vi "S4GUI_001.vi"() -> ()   [LabVIEW 2018] (continued)
        n2695 = call-dynamic "Write Kinetic Series Length.vi"("error in (no error)"=w6553, "Kinetic Series Length"=w6544, "Interface in"=w6554) -> ("error out"=w6545:errorcluster, "Interface out"=w6546:refnum<class "Interface.lvclass">)  [unwired: 7 in]
        n2696 = call-dynamic "Write Interface.vi"("error in (no error)"=w6545, "Interface.lvclass"=w6546, "Channel in"=w6552) -> ("error out"=w6551:errorcluster, "Channel out"=w6550:refnum<class "Channel.lvclass">)  [unwired: 7 in]
        n2697 = call-dynamic "Write Channel.vi"("error in (no error)"=w6551, "Channel.lvclass"=w6550, "Acquisition in"=w6549) -> ("error out"=w6555:errorcluster, "Acquisition out"=w6557:refnum<class "Acquisition.lvclass">)  [unwired: 7 in]
        n2698 = call-dynamic "Write AcquisitionA.vi"("error in (no error)"=w6555, "Acquisition.lvclass"=w6557, "S4ACS_GUI in"=w6556) -> ("error out"=w6541:errorcluster, "S4ACS_GUI out"=w6540:refnum<class "S4GUI.lvclass">)  [unwired: 7 in]
      }
      event "Stop ch1": Value Change {
        n2699 = event-data() -> ()  [unwired: 1 in, 6 out]
        n2700 = disable-structure shown="Enabled" {
          disable-tunnel: w6563 -> [w6596 w6624]
          disable-tunnel: w6562 -> [w6594 w6617]
          disable-tunnel: [w6576 w6616] -> w6561
          disable-tunnel: [w6564 w6624] -> w6560
          frame Disabled {
            # "Para movimento \nda lamina retardadora"
            # "Restaura a última sequência de lâminas"
            n2701 = call-dynamic "Read AcquisitionA.vi"("error in (no error)"=w6594, "S4ACS_GUI in"=w6596) -> ("error out"=w6598:errorcluster, "Acquisition.lvclass"=w6597:refnum<class "Acquisition.lvclass">, "S4ACS_GUI out"=w6595:refnum<class "S4GUI.lvclass">)  [unwired: 7 in]
            n2702 = disable-structure shown="Enabled" {
              disable-tunnel: w6598 -> [w6603 w6614]
              disable-tunnel: w6597 -> [w6602 w6615]
              disable-tunnel: [w6600 w6615] -> w6592
              disable-tunnel: [w6599 w6614] -> w6591
              frame Disabled {
                # "Só precisa enviar comando STOP quando\no controle dos ciclos for feito pelo ACS."
                n2703 = call-dynamic "Read Channel.vi"("error in (no error)"=w6603, "Acquisition in"=w6602) -> ("error out"=w6605:errorcluster, "Channel.lvclass"=w6604:refnum<class "Channel.lvclass">, "Acquisition out"=w6611:refnum<class "Acquisition.lvclass">)  [unwired: 7 in]
                n2704 = call-dynamic "Read State Machine.vi"("error in (no error)"=w6605, "Device in"=w6604) -> ("error out"=w6607:errorcluster, "State Machine.lvclass"=w6606:refnum<class "State Machine.lvclass">, "Device out"=w6609:refnum<class "Channel.lvclass">)  [unwired: 7 in]
                n2705 = call "Next State.vi"("error in (no error)"=w6607, "New_State"=u32 70, "State Machine in"=w6606) -> ("error out"=w6610:errorcluster, "State Machine out"=w6608:refnum<class "State Machine.lvclass">)  [unwired: 7 in]
                n2706 = call-dynamic "Write State Machine.vi"("error in (no error)"=w6610, "State Machine.lvclass"=w6608, "Device in"=w6609) -> ("error out"=w6612:errorcluster, "Device out"=w6613:refnum<class "Channel.lvclass">)  [unwired: 7 in]
                n2707 = call-dynamic "Write Channel.vi"("error in (no error)"=w6612, "Channel.lvclass"=w6613, "Acquisition in"=w6611) -> ("error out"=w6599:errorcluster, "Acquisition out"=w6600:refnum<class "Acquisition.lvclass">)  [unwired: 7 in]
              }
              frame Enabled {
                # "Não precisa enviar comando STOP para o ACS\nenquanto o controle dos ciclos for feito pela GUI."
              }
            }
            n2708 = call-dynamic "Write Acq_state.vi"("error in (no error)"=w6591, "Acq_state"=u32 0, "Acquisition in"=w6592) -> ("error out"=w6590:errorcluster, "Acquisition out"=w6589:refnum<class "Acquisition.lvclass">)  [unwired: 7 in]
            n2709 = call-dynamic "Write AcquisitionA.vi"("error in (no error)"=w6590, "Acquisition.lvclass"=w6589, "S4ACS_GUI in"=w6595) -> ("error out"=w6577:errorcluster, "S4ACS_GUI out"=w6575:refnum<class "S4GUI.lvclass">)  [unwired: 7 in]
            n2710 = call "Read Instrument.lvclass.vi"("error in (no error)"=w6577, "S4ACS_GUI in"=w6575) -> ("error out"=w6584:errorcluster, "Instrument.lvclass"=w6587:refnum<class "Instrument.lvclass">, "S4ACS_GUI out"=w6588:refnum<class "S4GUI.lvclass">)  [unwired: 7 in]
            n2711 = call "Read WPROT.vi"("error in (no error)"=w6584, "Instrument in"=w6587) -> ("error out"=w6583:errorcluster, "Opt_Selector.lvclass"=w6585:refnum<class "Opt_Selector.lvclass">, "Instrument out"=w6586:refnum<class "Instrument.lvclass">)  [unwired: 7 in]
            n2712 = call-dynamic "Read sequencia_ant.vi"("error in (no error)"=w6583, "Opt_Selector in"=w6585) -> ("error out"=w6579:errorcluster, "sequencia_ant"=w6578:u16, "Opt_Selector out"=w6580:refnum<class "Opt_Selector.lvclass">)  [unwired: 7 in]
            n2713 = call-dynamic "Write sequencia.vi"("error in (no error)"=w6579, "sequencia"=w6578, "Opt_Selector in"=w6580) -> ("error out"=w6566:errorcluster, "Opt_Selector out"=w6569:refnum<class "Opt_Selector.lvclass">)  [unwired: 7 in]
            n2714 = call-dynamic "Read State Machine.vi"("error in (no error)"=w6566, "Device in"=w6569) -> ("error out"=w6571:errorcluster, "State Machine.lvclass"=w6574:refnum<class "State Machine.lvclass">, "Device out"=w6568:refnum<class "Opt_Selector.lvclass">)  [unwired: 7 in]
            n2715 = call "Next State.vi"("error in (no error)"=w6571, "New_State"=10, "State Machine in"=w6574) -> ("error out"=w6570:errorcluster, "State Machine out"=w6573:refnum<class "State Machine.lvclass">)  [unwired: 7 in]
            n2716 = call-dynamic "Write State Machine.vi"("error in (no error)"=w6570, "State Machine.lvclass"=w6573, "Device in"=w6568) -> ("error out"=w6565:errorcluster, "Device out"=w6567:refnum<class "Opt_Selector.lvclass">)  [unwired: 7 in]
            n2717 = call "Write WPROT.vi"("error in (no error)"=w6565, "Opt_Selector.lvclass"=w6567, "Instrument in"=w6586) -> ("error out"=w6582:errorcluster, "Instrument out"=w6581:refnum<class "Instrument.lvclass">)  [unwired: 7 in]
            n2718 = call "Write Instrument.lvclass.vi"("error in (no error)"=w6582, "Instrument.lvclass"=w6581, "S4ACS_GUI in"=w6588) -> ("error out"=w6576:errorcluster, "S4ACS_GUI out"=w6564:refnum<class "S4GUI.lvclass">)  [unwired: 7 in]
          }
          frame Enabled {
            w6619 = FALSE ("Wait Until Done")
            n2719 = call <vilib>:"Application Directory.vi"() -> ("Application Directory"=w6622:path)
            n2720 = Build Path(base path=w6622, name or relative path="MsgStop1.vi") -> (appended path=w6623:path)
            n2721 = Open VI Reference(vi path=w6623, error in (no error)=w6617) -> (vi reference=w6621:refnum<vi>, error out=w6620:errorcluster)  [unwired: 4 in]
            n2722 = invoke class="VI" method="Run VI"(reference=w6621, error in=w6620, "Wait until done"=w6619, "Auto Dispose Ref"=w6619) -> (error out=w6616:errorcluster)  [unwired: 1 in, 4 out]
          }
        }
      }
      event "Stop ch2": Value Change {
        n2723 = event-data() -> ()  [unwired: 1 in, 6 out]
        n2724 = disable-structure shown="Enabled" {
          disable-tunnel: w6628 -> [w6661 w6681]
          disable-tunnel: w6627 -> [w6659 w6683]
          disable-tunnel: [w6641 w6682] -> w6626
          disable-tunnel: [w6629 w6681] -> w6625
          frame Disabled {
            # "Para movimento \nda lamina retardadora"
            # "Restaura a última sequência de lâminas"
            n2725 = call "Read AcquisitionB.vi"("error in (no error)"=w6659, "S4ACS_GUI in"=w6661) -> ("error out"=w6663:errorcluster, "Acquisition.lvclass"=w6662:refnum<class "Acquisition.lvclass">, "S4ACS_GUI out"=w6660:refnum<class "S4GUI.lvclass">)  [unwired: 7 in]
            n2726 = disable-structure shown="Enabled" {
              disable-tunnel: w6663 -> [w6668 w6679]
              disable-tunnel: w6662 -> [w6667 w6680]
              disable-tunnel: [w6665 w6680] -> w6657
              disable-tunnel: [w6664 w6679] -> w6656
              frame Disabled {
                # "Só precisa enviar comando STOP quando\no controle dos ciclos for feito pelo ACS."
                n2727 = call-dynamic "Read Channel.vi"("error in (no error)"=w6668, "Acquisition in"=w6667) -> ("error out"=w6670:errorcluster, "Channel.lvclass"=w6669:refnum<class "Channel.lvclass">, "Acquisition out"=w6676:refnum<class "Acquisition.lvclass">)  [unwired: 7 in]
                n2728 = call-dynamic "Read State Machine.vi"("error in (no error)"=w6670, "Device in"=w6669) -> ("error out"=w6672:errorcluster, "State Machine.lvclass"=w6671:refnum<class "State Machine.lvclass">, "Device out"=w6674:refnum<class "Channel.lvclass">)  [unwired: 7 in]
                n2729 = call "Next State.vi"("error in (no error)"=w6672, "New_State"=u32 70, "State Machine in"=w6671) -> ("error out"=w6675:errorcluster, "State Machine out"=w6673:refnum<class "State Machine.lvclass">)  [unwired: 7 in]
                n2730 = call-dynamic "Write State Machine.vi"("error in (no error)"=w6675, "State Machine.lvclass"=w6673, "Device in"=w6674) -> ("error out"=w6677:errorcluster, "Device out"=w6678:refnum<class "Channel.lvclass">)  [unwired: 7 in]
                n2731 = call-dynamic "Write Channel.vi"("error in (no error)"=w6677, "Channel.lvclass"=w6678, "Acquisition in"=w6676) -> ("error out"=w6664:errorcluster, "Acquisition out"=w6665:refnum<class "Acquisition.lvclass">)  [unwired: 7 in]
              }
              frame Enabled {
                # "Não precisa enviar comando STOP para o ACS\nenquanto o controle dos ciclos for feito pela GUI."
              }
            }
            n2732 = call-dynamic "Write Acq_state.vi"("error in (no error)"=w6656, "Acq_state"=u32 0, "Acquisition in"=w6657) -> ("error out"=w6655:errorcluster, "Acquisition out"=w6654:refnum<class "Acquisition.lvclass">)  [unwired: 7 in]
            n2733 = call "Write AcquisitionB.vi"("error in (no error)"=w6655, "Acquisition.lvclass"=w6654, "S4ACS_GUI in"=w6660) -> ("error out"=w6642:errorcluster, "S4ACS_GUI out"=w6640:refnum<class "S4GUI.lvclass">)  [unwired: 7 in]
            n2734 = call "Read Instrument.lvclass.vi"("error in (no error)"=w6642, "S4ACS_GUI in"=w6640) -> ("error out"=w6649:errorcluster, "Instrument.lvclass"=w6652:refnum<class "Instrument.lvclass">, "S4ACS_GUI out"=w6653:refnum<class "S4GUI.lvclass">)  [unwired: 7 in]
            n2735 = call "Read WPROT.vi"("error in (no error)"=w6649, "Instrument in"=w6652) -> ("error out"=w6648:errorcluster, "Opt_Selector.lvclass"=w6650:refnum<class "Opt_Selector.lvclass">, "Instrument out"=w6651:refnum<class "Instrument.lvclass">)  [unwired: 7 in]
            n2736 = call-dynamic "Read sequencia_ant.vi"("error in (no error)"=w6648, "Opt_Selector in"=w6650) -> ("error out"=w6644:errorcluster, "sequencia_ant"=w6643:u16, "Opt_Selector out"=w6645:refnum<class "Opt_Selector.lvclass">)  [unwired: 7 in]
            n2737 = call-dynamic "Write sequencia.vi"("error in (no error)"=w6644, "sequencia"=w6643, "Opt_Selector in"=w6645) -> ("error out"=w6631:errorcluster, "Opt_Selector out"=w6634:refnum<class "Opt_Selector.lvclass">)  [unwired: 7 in]
            n2738 = call-dynamic "Read State Machine.vi"("error in (no error)"=w6631, "Device in"=w6634) -> ("error out"=w6636:errorcluster, "State Machine.lvclass"=w6639:refnum<class "State Machine.lvclass">, "Device out"=w6633:refnum<class "Opt_Selector.lvclass">)  [unwired: 7 in]
            n2739 = call "Next State.vi"("error in (no error)"=w6636, "New_State"=10, "State Machine in"=w6639) -> ("error out"=w6635:errorcluster, "State Machine out"=w6638:refnum<class "State Machine.lvclass">)  [unwired: 7 in]
            n2740 = call-dynamic "Write State Machine.vi"("error in (no error)"=w6635, "State Machine.lvclass"=w6638, "Device in"=w6633) -> ("error out"=w6630:errorcluster, "Device out"=w6632:refnum<class "Opt_Selector.lvclass">)  [unwired: 7 in]
            n2741 = call "Write WPROT.vi"("error in (no error)"=w6630, "Opt_Selector.lvclass"=w6632, "Instrument in"=w6651) -> ("error out"=w6647:errorcluster, "Instrument out"=w6646:refnum<class "Instrument.lvclass">)  [unwired: 7 in]
            n2742 = call "Write Instrument.lvclass.vi"("error in (no error)"=w6647, "Instrument.lvclass"=w6646, "S4ACS_GUI in"=w6653) -> ("error out"=w6641:errorcluster, "S4ACS_GUI out"=w6629:refnum<class "S4GUI.lvclass">)  [unwired: 7 in]
          }
          frame Enabled {
            w6685 = FALSE ("Wait Until Done")
            n2743 = call <vilib>:"Application Directory.vi"() -> ("Application Directory"=w6688:path)
            n2744 = Build Path(base path=w6688, name or relative path="MsgStop2.vi") -> (appended path=w6689:path)
            n2745 = Open VI Reference(vi path=w6689, error in (no error)=w6683) -> (vi reference=w6687:refnum<vi>, error out=w6686:errorcluster)  [unwired: 4 in]
            n2746 = invoke class="VI" method="Run VI"(reference=w6687, error in=w6686, "Wait until done"=w6685, "Auto Dispose Ref"=w6685) -> (error out=w6682:errorcluster)  [unwired: 1 in, 4 out]
          }
        }
      }
      event "Stop ch3": Value Change {
        n2747 = event-data() -> ()  [unwired: 1 in, 6 out]
        n2748 = disable-structure shown="Enabled" {
          disable-tunnel: w6693 -> [w6726 w6746]
          disable-tunnel: w6692 -> [w6724 w6748]
          disable-tunnel: [w6706 w6747] -> w6691
          disable-tunnel: [w6694 w6746] -> w6690
          frame Disabled {
            # "Para movimento \nda lamina retardadora"
            # "Restaura a última sequência de lâminas"
            n2749 = call-dynamic "Read AcquisitionC.vi"("error in (no error)"=w6724, "S4ACS_GUI in"=w6726) -> ("error out"=w6728:errorcluster, "Acquisition.lvclass"=w6727:refnum<class "Acquisition.lvclass">, "S4ACS_GUI out"=w6725:refnum<class "S4GUI.lvclass">)  [unwired: 7 in]
            n2750 = disable-structure shown="Enabled" {
              disable-tunnel: w6728 -> [w6733 w6744]
              disable-tunnel: w6727 -> [w6732 w6745]
              disable-tunnel: [w6730 w6745] -> w6722
              disable-tunnel: [w6729 w6744] -> w6721
              frame Disabled {
                # "Só precisa enviar comando STOP quando\no controle dos ciclos for feito pelo ACS."
                n2751 = call-dynamic "Read Channel.vi"("error in (no error)"=w6733, "Acquisition in"=w6732) -> ("error out"=w6735:errorcluster, "Channel.lvclass"=w6734:refnum<class "Channel.lvclass">, "Acquisition out"=w6741:refnum<class "Acquisition.lvclass">)  [unwired: 7 in]
                n2752 = call-dynamic "Read State Machine.vi"("error in (no error)"=w6735, "Device in"=w6734) -> ("error out"=w6737:errorcluster, "State Machine.lvclass"=w6736:refnum<class "State Machine.lvclass">, "Device out"=w6739:refnum<class "Channel.lvclass">)  [unwired: 7 in]
                n2753 = call "Next State.vi"("error in (no error)"=w6737, "New_State"=u32 70, "State Machine in"=w6736) -> ("error out"=w6740:errorcluster, "State Machine out"=w6738:refnum<class "State Machine.lvclass">)  [unwired: 7 in]
                n2754 = call-dynamic "Write State Machine.vi"("error in (no error)"=w6740, "State Machine.lvclass"=w6738, "Device in"=w6739) -> ("error out"=w6742:errorcluster, "Device out"=w6743:refnum<class "Channel.lvclass">)  [unwired: 7 in]
                n2755 = call-dynamic "Write Channel.vi"("error in (no error)"=w6742, "Channel.lvclass"=w6743, "Acquisition in"=w6741) -> ("error out"=w6729:errorcluster, "Acquisition out"=w6730:refnum<class "Acquisition.lvclass">)  [unwired: 7 in]
              }
              frame Enabled {
                # "Não precisa enviar comando STOP para o ACS\nenquanto o controle dos ciclos for feito pela GUI."
              }
            }
            n2756 = call-dynamic "Write Acq_state.vi"("error in (no error)"=w6721, "Acq_state"=u32 0, "Acquisition in"=w6722) -> ("error out"=w6720:errorcluster, "Acquisition out"=w6719:refnum<class "Acquisition.lvclass">)  [unwired: 7 in]
            n2757 = call-dynamic "Write AcquisitionC.vi"("error in (no error)"=w6720, "Acquisition.lvclass"=w6719, "S4ACS_GUI in"=w6725) -> ("error out"=w6707:errorcluster, "S4ACS_GUI out"=w6705:refnum<class "S4GUI.lvclass">)  [unwired: 7 in]
            n2758 = call "Read Instrument.lvclass.vi"("error in (no error)"=w6707, "S4ACS_GUI in"=w6705) -> ("error out"=w6714:errorcluster, "Instrument.lvclass"=w6717:refnum<class "Instrument.lvclass">, "S4ACS_GUI out"=w6718:refnum<class "S4GUI.lvclass">)  [unwired: 7 in]
            n2759 = call "Read WPROT.vi"("error in (no error)"=w6714, "Instrument in"=w6717) -> ("error out"=w6713:errorcluster, "Opt_Selector.lvclass"=w6715:refnum<class "Opt_Selector.lvclass">, "Instrument out"=w6716:refnum<class "Instrument.lvclass">)  [unwired: 7 in]
            n2760 = call-dynamic "Read sequencia_ant.vi"("error in (no error)"=w6713, "Opt_Selector in"=w6715) -> ("error out"=w6709:errorcluster, "sequencia_ant"=w6708:u16, "Opt_Selector out"=w6710:refnum<class "Opt_Selector.lvclass">)  [unwired: 7 in]
            n2761 = call-dynamic "Write sequencia.vi"("error in (no error)"=w6709, "sequencia"=w6708, "Opt_Selector in"=w6710) -> ("error out"=w6696:errorcluster, "Opt_Selector out"=w6699:refnum<class "Opt_Selector.lvclass">)  [unwired: 7 in]
            n2762 = call-dynamic "Read State Machine.vi"("error in (no error)"=w6696, "Device in"=w6699) -> ("error out"=w6701:errorcluster, "State Machine.lvclass"=w6704:refnum<class "State Machine.lvclass">, "Device out"=w6698:refnum<class "Opt_Selector.lvclass">)  [unwired: 7 in]
            n2763 = call "Next State.vi"("error in (no error)"=w6701, "New_State"=10, "State Machine in"=w6704) -> ("error out"=w6700:errorcluster, "State Machine out"=w6703:refnum<class "State Machine.lvclass">)  [unwired: 7 in]
            n2764 = call-dynamic "Write State Machine.vi"("error in (no error)"=w6700, "State Machine.lvclass"=w6703, "Device in"=w6698) -> ("error out"=w6695:errorcluster, "Device out"=w6697:refnum<class "Opt_Selector.lvclass">)  [unwired: 7 in]
            n2765 = call "Write WPROT.vi"("error in (no error)"=w6695, "Opt_Selector.lvclass"=w6697, "Instrument in"=w6716) -> ("error out"=w6712:errorcluster, "Instrument out"=w6711:refnum<class "Instrument.lvclass">)  [unwired: 7 in]
            n2766 = call "Write Instrument.lvclass.vi"("error in (no error)"=w6712, "Instrument.lvclass"=w6711, "S4ACS_GUI in"=w6718) -> ("error out"=w6706:errorcluster, "S4ACS_GUI out"=w6694:refnum<class "S4GUI.lvclass">)  [unwired: 7 in]
          }
          frame Enabled {
            w6750 = FALSE ("Wait Until Done")
            n2767 = call <vilib>:"Application Directory.vi"() -> ("Application Directory"=w6753:path)
            n2768 = Build Path(base path=w6753, name or relative path="MsgStop3.vi") -> (appended path=w6754:path)
            n2769 = Open VI Reference(vi path=w6754, error in (no error)=w6748) -> (vi reference=w6752:refnum<vi>, error out=w6751:errorcluster)  [unwired: 4 in]
            n2770 = invoke class="VI" method="Run VI"(reference=w6752, error in=w6751, "Wait until done"=w6750, "Auto Dispose Ref"=w6750) -> (error out=w6747:errorcluster)  [unwired: 1 in, 4 out]
          }
        }
      }
      event "Stop ch4": Value Change {
        n2771 = event-data() -> ()  [unwired: 1 in, 6 out]
        n2772 = disable-structure shown="Enabled" {
          disable-tunnel: w6758 -> [w6791 w6811]
          disable-tunnel: w6757 -> [w6789 w6813]
          disable-tunnel: [w6771 w6812] -> w6756
          disable-tunnel: [w6759 w6811] -> w6755
          frame Disabled {
            # "Para movimento \nda lamina retardadora"
            # "Restaura a última sequência de lâminas"
            n2773 = call-dynamic "Read AcquisitionD.vi"("error in (no error)"=w6789, "S4ACS_GUI in"=w6791) -> ("error out"=w6793:errorcluster, "Acquisition.lvclass"=w6792:refnum<class "Acquisition.lvclass">, "S4ACS_GUI out"=w6790:refnum<class "S4GUI.lvclass">)  [unwired: 7 in]
            n2774 = disable-structure shown="Enabled" {
              disable-tunnel: w6793 -> [w6798 w6809]
              disable-tunnel: w6792 -> [w6797 w6810]
              disable-tunnel: [w6795 w6810] -> w6787
              disable-tunnel: [w6794 w6809] -> w6786
              frame Disabled {
                # "Só precisa enviar comando STOP quando\no controle dos ciclos for feito pelo ACS."
                n2775 = call-dynamic "Read Channel.vi"("error in (no error)"=w6798, "Acquisition in"=w6797) -> ("error out"=w6800:errorcluster, "Channel.lvclass"=w6799:refnum<class "Channel.lvclass">, "Acquisition out"=w6806:refnum<class "Acquisition.lvclass">)  [unwired: 7 in]
                n2776 = call-dynamic "Read State Machine.vi"("error in (no error)"=w6800, "Device in"=w6799) -> ("error out"=w6802:errorcluster, "State Machine.lvclass"=w6801:refnum<class "State Machine.lvclass">, "Device out"=w6804:refnum<class "Channel.lvclass">)  [unwired: 7 in]
                n2777 = call "Next State.vi"("error in (no error)"=w6802, "New_State"=u32 70, "State Machine in"=w6801) -> ("error out"=w6805:errorcluster, "State Machine out"=w6803:refnum<class "State Machine.lvclass">)  [unwired: 7 in]
                n2778 = call-dynamic "Write State Machine.vi"("error in (no error)"=w6805, "State Machine.lvclass"=w6803, "Device in"=w6804) -> ("error out"=w6807:errorcluster, "Device out"=w6808:refnum<class "Channel.lvclass">)  [unwired: 7 in]
                n2779 = call-dynamic "Write Channel.vi"("error in (no error)"=w6807, "Channel.lvclass"=w6808, "Acquisition in"=w6806) -> ("error out"=w6794:errorcluster, "Acquisition out"=w6795:refnum<class "Acquisition.lvclass">)  [unwired: 7 in]
              }
              frame Enabled {
                # "Não precisa enviar comando STOP para o ACS\nenquanto o controle dos ciclos for feito pela GUI."
              }
            }
            n2780 = call-dynamic "Write Acq_state.vi"("error in (no error)"=w6786, "Acq_state"=u32 0, "Acquisition in"=w6787) -> ("error out"=w6785:errorcluster, "Acquisition out"=w6784:refnum<class "Acquisition.lvclass">)  [unwired: 7 in]
            n2781 = call-dynamic "Write AcquisitionD.vi"("error in (no error)"=w6785, "Acquisition.lvclass"=w6784, "S4ACS_GUI in"=w6790) -> ("error out"=w6772:errorcluster, "S4ACS_GUI out"=w6770:refnum<class "S4GUI.lvclass">)  [unwired: 7 in]
            n2782 = call "Read Instrument.lvclass.vi"("error in (no error)"=w6772, "S4ACS_GUI in"=w6770) -> ("error out"=w6779:errorcluster, "Instrument.lvclass"=w6782:refnum<class "Instrument.lvclass">, "S4ACS_GUI out"=w6783:refnum<class "S4GUI.lvclass">)  [unwired: 7 in]
            n2783 = call "Read WPROT.vi"("error in (no error)"=w6779, "Instrument in"=w6782) -> ("error out"=w6778:errorcluster, "Opt_Selector.lvclass"=w6780:refnum<class "Opt_Selector.lvclass">, "Instrument out"=w6781:refnum<class "Instrument.lvclass">)  [unwired: 7 in]
            n2784 = call-dynamic "Read sequencia_ant.vi"("error in (no error)"=w6778, "Opt_Selector in"=w6780) -> ("error out"=w6774:errorcluster, "sequencia_ant"=w6773:u16, "Opt_Selector out"=w6775:refnum<class "Opt_Selector.lvclass">)  [unwired: 7 in]
            n2785 = call-dynamic "Write sequencia.vi"("error in (no error)"=w6774, "sequencia"=w6773, "Opt_Selector in"=w6775) -> ("error out"=w6761:errorcluster, "Opt_Selector out"=w6764:refnum<class "Opt_Selector.lvclass">)  [unwired: 7 in]
            n2786 = call-dynamic "Read State Machine.vi"("error in (no error)"=w6761, "Device in"=w6764) -> ("error out"=w6766:errorcluster, "State Machine.lvclass"=w6769:refnum<class "State Machine.lvclass">, "Device out"=w6763:refnum<class "Opt_Selector.lvclass">)  [unwired: 7 in]
            n2787 = call "Next State.vi"("error in (no error)"=w6766, "New_State"=10, "State Machine in"=w6769) -> ("error out"=w6765:errorcluster, "State Machine out"=w6768:refnum<class "State Machine.lvclass">)  [unwired: 7 in]
            n2788 = call-dynamic "Write State Machine.vi"("error in (no error)"=w6765, "State Machine.lvclass"=w6768, "Device in"=w6763) -> ("error out"=w6760:errorcluster, "Device out"=w6762:refnum<class "Opt_Selector.lvclass">)  [unwired: 7 in]
            n2789 = call "Write WPROT.vi"("error in (no error)"=w6760, "Opt_Selector.lvclass"=w6762, "Instrument in"=w6781) -> ("error out"=w6777:errorcluster, "Instrument out"=w6776:refnum<class "Instrument.lvclass">)  [unwired: 7 in]
            n2790 = call "Write Instrument.lvclass.vi"("error in (no error)"=w6777, "Instrument.lvclass"=w6776, "S4ACS_GUI in"=w6783) -> ("error out"=w6771:errorcluster, "S4ACS_GUI out"=w6759:refnum<class "S4GUI.lvclass">)  [unwired: 7 in]
          }
          frame Enabled {
            w6815 = FALSE ("Wait Until Done")
            n2791 = call <vilib>:"Application Directory.vi"() -> ("Application Directory"=w6818:path)
            n2792 = Build Path(base path=w6818, name or relative path="MsgStop4.vi") -> (appended path=w6819:path)
            n2793 = Open VI Reference(vi path=w6819, error in (no error)=w6813) -> (vi reference=w6817:refnum<vi>, error out=w6816:errorcluster)  [unwired: 4 in]
            n2794 = invoke class="VI" method="Run VI"(reference=w6817, error in=w6816, "Wait until done"=w6815, "Auto Dispose Ref"=w6815) -> (error out=w6812:errorcluster)  [unwired: 1 in, 4 out]
          }
        }
      }
      event "Pause ch1": Value Change {
        n2795 = event-data() -> ()  [unwired: 1 in, 6 out]
        n2796 = disable-structure shown="Enabled" {
          disable-tunnel: w6823 -> [w6839 w6850]
          disable-tunnel: [w6837 w6848] -> w6822
          disable-tunnel: w6821 -> [w6836 w6849]
          disable-tunnel: [w6824 w6850] -> w6820
          frame Disabled {
            n2797 = call-dynamic "Read AcquisitionA.vi"("error in (no error)"=w6836, "S4ACS_GUI in"=w6839) -> ("error out"=w6831:errorcluster, "Acquisition.lvclass"=w6830:refnum<class "Acquisition.lvclass">, "S4ACS_GUI out"=w6838:refnum<class "S4GUI.lvclass">)  [unwired: 7 in]
            n2798 = call-dynamic "Read Acq_state.vi"("error in (no error)"=w6831, "Acquisition in"=w6830) -> ("error out"=w6833:errorcluster, "Acq_state"=w6834:u32, "Acquisition out"=w6835:refnum<class "Acquisition.lvclass">)  [unwired: 7 in]
            n2799 = call-dynamic "Write Acq_prevstate.vi"("error in (no error)"=w6833, "Acq_prevstate"=w6834, "Acquisition in"=w6835) -> ("error out"=w6828:errorcluster, "Acquisition out"=w6829:refnum<class "Acquisition.lvclass">)  [unwired: 7 in]
            n2800 = call-dynamic "Write Acq_state.vi"("error in (no error)"=w6828, "Acq_state"=u32 400, "Acquisition in"=w6829) -> ("error out"=w6826:errorcluster, "Acquisition out"=w6827:refnum<class "Acquisition.lvclass">)  [unwired: 7 in]
            n2801 = disable-structure shown="Enabled" {
              disable-tunnel: w6826 -> [w6841 w6847]
              disable-tunnel: [w6840 w6847] -> w6825
              frame Disabled {
                n2802 = property on="Start ch1" class="Bool"(error in=w6841, "BoolText.Text"="RESUME" ("Caption.Text")) -> (error out=w6845:errorcluster)  [unwired: 1 in, 1 out]
                n2803 = property on="Pause ch1" class="Bool"(error in=w6845, "DisabledEnum"=T7."Disabled and Grayed Out" ("Disabled")) -> (error out=w6846:errorcluster)  [unwired: 1 in, 1 out]
                n2804 = property on="Start ch1" class="Bool"(error in=w6846, "DisabledEnum"=T7."Enabled" ("Disabled")) -> (error out=w6840:errorcluster)  [unwired: 1 in, 1 out]
              }
              frame Enabled {
              }
            }
            n2805 = call-dynamic "Write AcquisitionA.vi"("error in (no error)"=w6825, "Acquisition.lvclass"=w6827, "S4ACS_GUI in"=w6838) -> ("error out"=w6837:errorcluster, "S4ACS_GUI out"=w6824:refnum<class "S4GUI.lvclass">)  [unwired: 7 in]
          }
          frame Enabled {
            w6852 = FALSE ("Wait Until Done")
            n2806 = call <vilib>:"Application Directory.vi"() -> ("Application Directory"=w6855:path)
            n2807 = Build Path(base path=w6855, name or relative path="MsgPause1.vi") -> (appended path=w6856:path)
            n2808 = Open VI Reference(vi path=w6856, error in (no error)=w6849) -> (vi reference=w6854:refnum<vi>, error out=w6853:errorcluster)  [unwired: 4 in]
            n2809 = invoke class="VI" method="Run VI"(reference=w6854, error in=w6853, "Wait until done"=w6852, "Auto Dispose Ref"=w6852) -> (error out=w6848:errorcluster)  [unwired: 1 in, 4 out]
          }
        }
      }
      event "Pause ch2": Value Change {
        n2810 = event-data() -> ()  [unwired: 1 in, 6 out]
        n2811 = disable-structure shown="Enabled" {
          disable-tunnel: w6860 -> [w6875 w6876]
          disable-tunnel: [w6873 w6877] -> w6859
          disable-tunnel: w6858 -> [w6872 w6878]
          disable-tunnel: [w6862 w6876] -> w6857
          frame Disabled {
            n2812 = call "Read AcquisitionB.vi"("error in (no error)"=w6872, "S4ACS_GUI in"=w6875) -> ("error out"=w6867:errorcluster, "Acquisition.lvclass"=w6866:refnum<class "Acquisition.lvclass">, "S4ACS_GUI out"=w6874:refnum<class "S4GUI.lvclass">)  [unwired: 7 in]
            n2813 = call-dynamic "Read Acq_state.vi"("error in (no error)"=w6867, "Acquisition in"=w6866) -> ("error out"=w6869:errorcluster, "Acq_state"=w6870:u32, "Acquisition out"=w6871:refnum<class "Acquisition.lvclass">)  [unwired: 7 in]
            n2814 = call-dynamic "Write Acq_prevstate.vi"("error in (no error)"=w6869, "Acq_prevstate"=w6870, "Acquisition in"=w6871) -> ("error out"=w6864:errorcluster, "Acquisition out"=w6865:refnum<class "Acquisition.lvclass">)  [unwired: 7 in]
            n2815 = call-dynamic "Write Acq_state.vi"("error in (no error)"=w6864, "Acq_state"=u32 400, "Acquisition in"=w6865) -> ("error out"=w6861:errorcluster, "Acquisition out"=w6863:refnum<class "Acquisition.lvclass">)  [unwired: 7 in]
            n2816 = call "Write AcquisitionB.vi"("error in (no error)"=w6861, "Acquisition.lvclass"=w6863, "S4ACS_GUI in"=w6874) -> ("error out"=w6873:errorcluster, "S4ACS_GUI out"=w6862:refnum<class "S4GUI.lvclass">)  [unwired: 7 in]
          }
          frame Enabled {
            w6880 = FALSE ("Wait Until Done")
            n2817 = call <vilib>:"Application Directory.vi"() -> ("Application Directory"=w6883:path)
            n2818 = Build Path(base path=w6883, name or relative path="MsgPause2.vi") -> (appended path=w6884:path)
            n2819 = Open VI Reference(vi path=w6884, error in (no error)=w6878) -> (vi reference=w6882:refnum<vi>, error out=w6881:errorcluster)  [unwired: 4 in]
            n2820 = invoke class="VI" method="Run VI"(reference=w6882, error in=w6881, "Wait until done"=w6880, "Auto Dispose Ref"=w6880) -> (error out=w6877:errorcluster)  [unwired: 1 in, 4 out]
          }
        }
      }
      event "Pause ch3": Value Change {
        n2821 = event-data() -> ()  [unwired: 1 in, 6 out]
        n2822 = disable-structure shown="Enabled" {
          disable-tunnel: w6888 -> [w6903 w6904]
          disable-tunnel: [w6901 w6905] -> w6887
          disable-tunnel: w6886 -> [w6900 w6906]
          disable-tunnel: [w6890 w6904] -> w6885
          frame Disabled {
            n2823 = call-dynamic "Read AcquisitionC.vi"("error in (no error)"=w6900, "S4ACS_GUI in"=w6903) -> ("error out"=w6895:errorcluster, "Acquisition.lvclass"=w6894:refnum<class "Acquisition.lvclass">, "S4ACS_GUI out"=w6902:refnum<class "S4GUI.lvclass">)  [unwired: 7 in]
            n2824 = call-dynamic "Read Acq_state.vi"("error in (no error)"=w6895, "Acquisition in"=w6894) -> ("error out"=w6897:errorcluster, "Acq_state"=w6898:u32, "Acquisition out"=w6899:refnum<class "Acquisition.lvclass">)  [unwired: 7 in]
            n2825 = call-dynamic "Write Acq_prevstate.vi"("error in (no error)"=w6897, "Acq_prevstate"=w6898, "Acquisition in"=w6899) -> ("error out"=w6892:errorcluster, "Acquisition out"=w6893:refnum<class "Acquisition.lvclass">)  [unwired: 7 in]
            n2826 = call-dynamic "Write Acq_state.vi"("error in (no error)"=w6892, "Acq_state"=u32 400, "Acquisition in"=w6893) -> ("error out"=w6889:errorcluster, "Acquisition out"=w6891:refnum<class "Acquisition.lvclass">)  [unwired: 7 in]
            n2827 = call-dynamic "Write AcquisitionC.vi"("error in (no error)"=w6889, "Acquisition.lvclass"=w6891, "S4ACS_GUI in"=w6902) -> ("error out"=w6901:errorcluster, "S4ACS_GUI out"=w6890:refnum<class "S4GUI.lvclass">)  [unwired: 7 in]
          }
          frame Enabled {
            w6908 = FALSE ("Wait Until Done")
            n2828 = call <vilib>:"Application Directory.vi"() -> ("Application Directory"=w6911:path)
            n2829 = Build Path(base path=w6911, name or relative path="MsgPause3.vi") -> (appended path=w6912:path)
            n2830 = Open VI Reference(vi path=w6912, error in (no error)=w6906) -> (vi reference=w6910:refnum<vi>, error out=w6909:errorcluster)  [unwired: 4 in]
            n2831 = invoke class="VI" method="Run VI"(reference=w6910, error in=w6909, "Wait until done"=w6908, "Auto Dispose Ref"=w6908) -> (error out=w6905:errorcluster)  [unwired: 1 in, 4 out]
          }
        }
      }
      event "Pause ch4": Value Change {
        n2832 = event-data() -> ()  [unwired: 1 in, 6 out]
        n2833 = disable-structure shown="Enabled" {
          disable-tunnel: w6916 -> [w6931 w6940]
          disable-tunnel: [w6929 w6932] -> w6915
          disable-tunnel: w6914 -> [w6928 w6933]
          disable-tunnel: [w6918 w6940] -> w6913
          frame Disabled {
            n2834 = call-dynamic "Read AcquisitionD.vi"("error in (no error)"=w6928, "S4ACS_GUI in"=w6931) -> ("error out"=w6923:errorcluster, "Acquisition.lvclass"=w6922:refnum<class "Acquisition.lvclass">, "S4ACS_GUI out"=w6930:refnum<class "S4GUI.lvclass">)  [unwired: 7 in]
            n2835 = call-dynamic "Read Acq_state.vi"("error in (no error)"=w6923, "Acquisition in"=w6922) -> ("error out"=w6925:errorcluster, "Acq_state"=w6926:u32, "Acquisition out"=w6927:refnum<class "Acquisition.lvclass">)  [unwired: 7 in]
            n2836 = call-dynamic "Write Acq_prevstate.vi"("error in (no error)"=w6925, "Acq_prevstate"=w6926, "Acquisition in"=w6927) -> ("error out"=w6920:errorcluster, "Acquisition out"=w6921:refnum<class "Acquisition.lvclass">)  [unwired: 7 in]
            n2837 = call-dynamic "Write Acq_state.vi"("error in (no error)"=w6920, "Acq_state"=u32 400, "Acquisition in"=w6921) -> ("error out"=w6917:errorcluster, "Acquisition out"=w6919:refnum<class "Acquisition.lvclass">)  [unwired: 7 in]
            n2838 = call-dynamic "Write AcquisitionD.vi"("error in (no error)"=w6917, "Acquisition.lvclass"=w6919, "S4ACS_GUI in"=w6930) -> ("error out"=w6929:errorcluster, "S4ACS_GUI out"=w6918:refnum<class "S4GUI.lvclass">)  [unwired: 7 in]
          }
          frame Enabled {
            w6935 = FALSE ("Wait Until Done")
            n2839 = call <vilib>:"Application Directory.vi"() -> ("Application Directory"=w6938:path)
            n2840 = Build Path(base path=w6938, name or relative path="MsgPause4.vi") -> (appended path=w6939:path)
            n2841 = Open VI Reference(vi path=w6939, error in (no error)=w6933) -> (vi reference=w6937:refnum<vi>, error out=w6936:errorcluster)  [unwired: 4 in]
            n2842 = invoke class="VI" method="Run VI"(reference=w6937, error in=w6936, "Wait until done"=w6935, "Auto Dispose Ref"=w6935) -> (error out=w6932:errorcluster)  [unwired: 1 in, 4 out]
          }
        }
      }
      event "Stop SM": Value Change {
        w6941 = 0.0 ("Scale.Range:Minor Increment")
        n2843 = event-data() -> ()  [unwired: 1 in, 6 out]
        n2844 = disable-structure shown="Enabled" {
          disable-tunnel: w6946 -> [w6980 w7003]
          disable-tunnel: w6945 -> [w6978 w7004]
          disable-tunnel: [w6965 w7002] -> w6943
          disable-tunnel: [w6949 w7003] -> w6942
          frame Disabled {
            # "Não precisa enviar comando STOP para o ACS\nenquanto o controle dos ciclos for feito pela GUI."
            # "Para movimento \nda lamina retardadora"
            # "Restaura a sequencia anterior"
            n2845 = call-dynamic "Read AcquisitionA.vi"("error in (no error)"=w6978, "S4ACS_GUI in"=w6980) -> ("error out"=w6982:errorcluster, "Acquisition.lvclass"=w6981:refnum<class "Acquisition.lvclass">, "S4ACS_GUI out"=w6979:refnum<class "S4GUI.lvclass">)  [unwired: 7 in]
            n2846 = disable-structure shown="Enabled" {
              disable-tunnel: [w6996 w7000] -> w6984
              disable-tunnel: [w6995 w7001] -> w6983
              disable-tunnel: w6982 -> [w6987 w7000]
              disable-tunnel: w6981 -> [w6986 w7001]
              frame Disabled {
                n2847 = call-dynamic "Read Channel.vi"("error in (no error)"=w6987, "Acquisition in"=w6986) -> ("error out"=w6989:errorcluster, "Channel.lvclass"=w6988:refnum<class "Channel.lvclass">, "Acquisition out"=w6997:refnum<class "Acquisition.lvclass">)  [unwired: 7 in]
                n2848 = call-dynamic "Read State Machine.vi"("error in (no error)"=w6989, "Device in"=w6988) -> ("error out"=w6991:errorcluster, "State Machine.lvclass"=w6990:refnum<class "State Machine.lvclass">, "Device out"=w6993:refnum<class "Channel.lvclass">)  [unwired: 7 in]
                n2849 = call "Next State.vi"("error in (no error)"=w6991, "New_State"=u32 70, "State Machine in"=w6990) -> ("error out"=w6994:errorcluster, "State Machine out"=w6992:refnum<class "State Machine.lvclass">)  [unwired: 7 in]
                n2850 = call-dynamic "Write State Machine.vi"("error in (no error)"=w6994, "State Machine.lvclass"=w6992, "Device in"=w6993) -> ("error out"=w6998:errorcluster, "Device out"=w6999:refnum<class "Channel.lvclass">)  [unwired: 7 in]
                n2851 = call-dynamic "Write Channel.vi"("error in (no error)"=w6998, "Channel.lvclass"=w6999, "Acquisition in"=w6997) -> ("error out"=w6996:errorcluster, "Acquisition out"=w6995:refnum<class "Acquisition.lvclass">)  [unwired: 7 in]
              }
              frame Enabled {
              }
            }
            n2852 = call-dynamic "Write AcquisitionA.vi"("error in (no error)"=w6984, "Acquisition.lvclass"=w6983, "S4ACS_GUI in"=w6979) -> ("error out"=w6947:errorcluster, "S4ACS_GUI out"=w6948:refnum<class "S4GUI.lvclass">)  [unwired: 7 in]
            n2853 = call-dynamic "Write Obs_state.vi"("error in (no error)"=w6947, "Obs_state"=u32 0, "S4ACS_GUI in"=w6948) -> ("error out"=w6967:errorcluster, "S4ACS_GUI out"=w6968:refnum<class "S4GUI.lvclass">)  [unwired: 7 in]
            n2854 = call "Read Instrument.lvclass.vi"("error in (no error)"=w6967, "S4ACS_GUI in"=w6968) -> ("error out"=w6976:errorcluster, "Instrument.lvclass"=w6974:refnum<class "Instrument.lvclass">, "S4ACS_GUI out"=w6975:refnum<class "S4GUI.lvclass">)  [unwired: 7 in]
            n2855 = call "Read WPROT.vi"("error in (no error)"=w6976, "Instrument in"=w6974) -> ("error out"=w6961:errorcluster, "Opt_Selector.lvclass"=w6964:refnum<class "Opt_Selector.lvclass">, "Instrument out"=w6973:refnum<class "Instrument.lvclass">)  [unwired: 7 in]
            n2856 = call-dynamic "Read sequencia_ant.vi"("error in (no error)"=w6961, "Opt_Selector in"=w6964) -> ("error out"=w6960:errorcluster, "sequencia_ant"=w6962:u16, "Opt_Selector out"=w6963:refnum<class "Opt_Selector.lvclass">)  [unwired: 7 in]
            n2857 = call-dynamic "Write sequencia.vi"("error in (no error)"=w6960, "sequencia"=w6962, "Opt_Selector in"=w6963) -> ("error out"=w6958:errorcluster, "Opt_Selector out"=w6959:refnum<class "Opt_Selector.lvclass">)  [unwired: 7 in]
            n2858 = call-dynamic "Read State Machine.vi"("error in (no error)"=w6958, "Device in"=w6959) -> ("error out"=w6953:errorcluster, "State Machine.lvclass"=w6956:refnum<class "State Machine.lvclass">, "Device out"=w6957:refnum<class "Opt_Selector.lvclass">)  [unwired: 7 in]
            n2859 = call "Next State.vi"("error in (no error)"=w6953, "New_State"=10, "State Machine in"=w6956) -> ("error out"=w6952:errorcluster, "State Machine out"=w6955:refnum<class "State Machine.lvclass">)  [unwired: 7 in]
            n2860 = call-dynamic "Write State Machine.vi"("error in (no error)"=w6952, "State Machine.lvclass"=w6955, "Device in"=w6957) -> ("error out"=w6951:errorcluster, "Device out"=w6950:refnum<class "Opt_Selector.lvclass">)  [unwired: 7 in]
            n2861 = call "Write WPROT.vi"("error in (no error)"=w6951, "Opt_Selector.lvclass"=w6950, "Instrument in"=w6973) -> ("error out"=w6971:errorcluster, "Instrument out"=w6972:refnum<class "Instrument.lvclass">)  [unwired: 7 in]
            n2862 = call "Write Instrument.lvclass.vi"("error in (no error)"=w6971, "Instrument.lvclass"=w6972, "S4ACS_GUI in"=w6975) -> ("error out"=w6970:errorcluster, "S4ACS_GUI out"=w6969:refnum<class "S4GUI.lvclass">)  [unwired: 7 in]
            n2863 = call-dynamic "Write ciclos.vi"("error in (no error)"=w6970, "ciclos"=u32 0, "S4ACS_GUI in"=w6969) -> ("error out"=w6965:errorcluster, "S4ACS_GUI out"=w6949:refnum<class "S4GUI.lvclass">)  [unwired: 7 in]
          }
          frame Enabled {
            w7006 = FALSE ("Wait Until Done")
            n2864 = call <vilib>:"Application Directory.vi"() -> ("Application Directory"=w7009:path)
            n2865 = Build Path(base path=w7009, name or relative path="MsgStopSync.vi") -> (appended path=w7010:path)
            n2866 = Open VI Reference(vi path=w7010, error in (no error)=w7004) -> (vi reference=w7008:refnum<vi>, error out=w7007:errorcluster)  [unwired: 4 in]
            n2867 = invoke class="VI" method="Run VI"(reference=w7008, error in=w7007, "Wait until done"=w7006, "Auto Dispose Ref"=w7006) -> (error out=w7002:errorcluster)  [unwired: 1 in, 4 out]
          }
        }
        n2868 = property on="#Cycles Done" class="Slide (strict)"(error in=w6943, "Scale.Maximum"=w6941, "Scale.Minimum"=w6941) -> (error out=w6944:errorcluster)  [unwired: 1 in, 1 out]
      }
      event "Abort SM": Value Change {
        w7013 = 0.0 ("Scale.Range:Minor Increment")
        n2869 = event-data() -> ()  [unwired: 1 in, 6 out]
        n2870 = disable-structure shown="Enabled" {
          disable-tunnel: w7016 -> [w7106 w7129]
          disable-tunnel: w7015 -> [w7104 w7131]
          disable-tunnel: [w7018 w7129] -> w7012
          disable-tunnel: [w7017 w7130] -> w7011
          frame Disabled {
            # "Restaura a sequencia anterior"
            # "Para movimento \nda lamina retardadora"
            n2871 = call-dynamic "Read AcquisitionA.vi"("error in (no error)"=w7104, "S4ACS_GUI in"=w7106) -> ("error out"=w7109:errorcluster, "Acquisition.lvclass"=w7108:refnum<class "Acquisition.lvclass">, "S4ACS_GUI out"=w7105:refnum<class "S4GUI.lvclass">)  [unwired: 7 in]
            n2872 = call-dynamic "Read Channel.vi"("error in (no error)"=w7109, "Acquisition in"=w7108) -> ("error out"=w7111:errorcluster, "Channel.lvclass"=w7110:refnum<class "Channel.lvclass">, "Acquisition out"=w7119:refnum<class "Acquisition.lvclass">)  [unwired: 7 in]
            n2873 = call-dynamic "Read State Machine.vi"("error in (no error)"=w7111, "Device in"=w7110) -> ("error out"=w7113:errorcluster, "State Machine.lvclass"=w7112:refnum<class "State Machine.lvclass">, "Device out"=w7115:refnum<class "Channel.lvclass">)  [unwired: 7 in]
            n2874 = call "Next State.vi"("error in (no error)"=w7113, "New_State"=u32 80, "State Machine in"=w7112) -> ("error out"=w7116:errorcluster, "State Machine out"=w7114:refnum<class "State Machine.lvclass">)  [unwired: 7 in]
            n2875 = call-dynamic "Write State Machine.vi"("error in (no error)"=w7116, "State Machine.lvclass"=w7114, "Device in"=w7115) -> ("error out"=w7120:errorcluster, "Device out"=w7121:refnum<class "Channel.lvclass">)  [unwired: 7 in]
            n2876 = call-dynamic "Write Channel.vi"("error in (no error)"=w7120, "Channel.lvclass"=w7121, "Acquisition in"=w7119) -> ("error out"=w7118:errorcluster, "Acquisition out"=w7117:refnum<class "Acquisition.lvclass">)  [unwired: 7 in]
            n2877 = call-dynamic "Write AcquisitionA.vi"("error in (no error)"=w7118, "Acquisition.lvclass"=w7117, "S4ACS_GUI in"=w7105) -> ("error out"=w7090:errorcluster, "S4ACS_GUI out"=w7089:refnum<class "S4GUI.lvclass">)  [unwired: 7 in]
            n2878 = call "Read AcquisitionB.vi"("error in (no error)"=w7090, "S4ACS_GUI in"=w7089) -> ("error out"=w7083:errorcluster, "Acquisition.lvclass"=w7087:refnum<class "Acquisition.lvclass">, "S4ACS_GUI out"=w7088:refnum<class "S4GUI.lvclass">)  [unwired: 7 in]
            n2879 = call-dynamic "Read Channel.vi"("error in (no error)"=w7083, "Acquisition in"=w7087) -> ("error out"=w7098:errorcluster, "Channel.lvclass"=w7099:refnum<class "Channel.lvclass">, "Acquisition out"=w7085:refnum<class "Acquisition.lvclass">)  [unwired: 7 in]
            n2880 = call-dynamic "Read State Machine.vi"("error in (no error)"=w7098, "Device in"=w7099) -> ("error out"=w7096:errorcluster, "State Machine.lvclass"=w7097:refnum<class "State Machine.lvclass">, "Device out"=w7094:refnum<class "Channel.lvclass">)  [unwired: 7 in]
            n2881 = call "Next State.vi"("error in (no error)"=w7096, "New_State"=u32 80, "State Machine in"=w7097) -> ("error out"=w7093:errorcluster, "State Machine out"=w7095:refnum<class "State Machine.lvclass">)  [unwired: 7 in]
            n2882 = call-dynamic "Write State Machine.vi"("error in (no error)"=w7093, "State Machine.lvclass"=w7095, "Device in"=w7094) -> ("error out"=w7092:errorcluster, "Device out"=w7091:refnum<class "Channel.lvclass">)  [unwired: 7 in]
            n2883 = call-dynamic "Write Channel.vi"("error in (no error)"=w7092, "Channel.lvclass"=w7091, "Acquisition in"=w7085) -> ("error out"=w7084:errorcluster, "Acquisition out"=w7086:refnum<class "Acquisition.lvclass">)  [unwired: 7 in]
            n2884 = call "Write AcquisitionB.vi"("error in (no error)"=w7084, "Acquisition.lvclass"=w7086, "S4ACS_GUI in"=w7088) -> ("error out"=w7050:errorcluster, "S4ACS_GUI out"=w7049:refnum<class "S4GUI.lvclass">)  [unwired: 7 in]
            n2885 = call-dynamic "Read AcquisitionC.vi"("error in (no error)"=w7050, "S4ACS_GUI in"=w7049) -> ("error out"=w7067:errorcluster, "Acquisition.lvclass"=w7071:refnum<class "Acquisition.lvclass">, "S4ACS_GUI out"=w7072:refnum<class "S4GUI.lvclass">)  [unwired: 7 in]
            n2886 = call-dynamic "Read Channel.vi"("error in (no error)"=w7067, "Acquisition in"=w7071) -> ("error out"=w7080:errorcluster, "Channel.lvclass"=w7081:refnum<class "Channel.lvclass">, "Acquisition out"=w7069:refnum<class "Acquisition.lvclass">)  [unwired: 7 in]
            n2887 = call-dynamic "Read State Machine.vi"("error in (no error)"=w7080, "Device in"=w7081) -> ("error out"=w7078:errorcluster, "State Machine.lvclass"=w7079:refnum<class "State Machine.lvclass">, "Device out"=w7076:refnum<class "Channel.lvclass">)  [unwired: 7 in]
            n2888 = call "Next State.vi"("error in (no error)"=w7078, "New_State"=u32 80, "State Machine in"=w7079) -> ("error out"=w7075:errorcluster, "State Machine out"=w7077:refnum<class "State Machine.lvclass">)  [unwired: 7 in]
            n2889 = call-dynamic "Write State Machine.vi"("error in (no error)"=w7075, "State Machine.lvclass"=w7077, "Device in"=w7076) -> ("error out"=w7074:errorcluster, "Device out"=w7073:refnum<class "Channel.lvclass">)  [unwired: 7 in]
            n2890 = call-dynamic "Write Channel.vi"("error in (no error)"=w7074, "Channel.lvclass"=w7073, "Acquisition in"=w7069) -> ("error out"=w7068:errorcluster, "Acquisition out"=w7070:refnum<class "Acquisition.lvclass">)  [unwired: 7 in]
            n2891 = call-dynamic "Write AcquisitionC.vi"("error in (no error)"=w7068, "Acquisition.lvclass"=w7070, "S4ACS_GUI in"=w7072) -> ("error out"=w7048:errorcluster, "S4ACS_GUI out"=w7047:refnum<class "S4GUI.lvclass">)  [unwired: 7 in]
            n2892 = call-dynamic "Read AcquisitionD.vi"("error in (no error)"=w7048, "S4ACS_GUI in"=w7047) -> ("error out"=w7051:errorcluster, "Acquisition.lvclass"=w7055:refnum<class "Acquisition.lvclass">, "S4ACS_GUI out"=w7056:refnum<class "S4GUI.lvclass">)  [unwired: 7 in]
            n2893 = call-dynamic "Read Channel.vi"("error in (no error)"=w7051, "Acquisition in"=w7055) -> ("error out"=w7064:errorcluster, "Channel.lvclass"=w7065:refnum<class "Channel.lvclass">, "Acquisition out"=w7053:refnum<class "Acquisition.lvclass">)  [unwired: 7 in]
            n2894 = call-dynamic "Read State Machine.vi"("error in (no error)"=w7064, "Device in"=w7065) -> ("error out"=w7062:errorcluster, "State Machine.lvclass"=w7063:refnum<class "State Machine.lvclass">, "Device out"=w7060:refnum<class "Channel.lvclass">)  [unwired: 7 in]
            n2895 = call "Next State.vi"("error in (no error)"=w7062, "New_State"=u32 80, "State Machine in"=w7063) -> ("error out"=w7059:errorcluster, "State Machine out"=w7061:refnum<class "State Machine.lvclass">)  [unwired: 7 in]
            n2896 = call-dynamic "Write State Machine.vi"("error in (no error)"=w7059, "State Machine.lvclass"=w7061, "Device in"=w7060) -> ("error out"=w7058:errorcluster, "Device out"=w7057:refnum<class "Channel.lvclass">)  [unwired: 7 in]
            n2897 = call-dynamic "Write Channel.vi"("error in (no error)"=w7058, "Channel.lvclass"=w7057, "Acquisition in"=w7053) -> ("error out"=w7052:errorcluster, "Acquisition out"=w7054:refnum<class "Acquisition.lvclass">)  [unwired: 7 in]
            n2898 = call-dynamic "Write AcquisitionD.vi"("error in (no error)"=w7052, "Acquisition.lvclass"=w7054, "S4ACS_GUI in"=w7056) -> ("error out"=w7045:errorcluster, "S4ACS_GUI out"=w7046:refnum<class "S4GUI.lvclass">)  [unwired: 7 in]
            n2899 = disable-structure shown="Enabled" {
              disable-tunnel: w7046 -> [w7126 w7128]
              disable-tunnel: w7045 -> [w7125 w7127]
              disable-tunnel: [w7123 w7128] -> w7102
              disable-tunnel: [w7122 w7127] -> w7101
              frame Disabled {
                n2900 = call-dynamic "Write aborted.vi"("error in (no error)"=w7125, "aborted"=TRUE ("stopped"), "S4ACS_GUI in"=w7126) -> ("error out"=w7122:errorcluster, "S4ACS_GUI out"=w7123:refnum<class "S4GUI.lvclass">)  [unwired: 7 in]
              }
              frame Enabled {
              }
            }
            n2901 = call-dynamic "Write Obs_state.vi"("error in (no error)"=w7101, "Obs_state"=u32 0, "S4ACS_GUI in"=w7102) -> ("error out"=w7019:errorcluster, "S4ACS_GUI out"=w7020:refnum<class "S4GUI.lvclass">)  [unwired: 7 in]
            n2902 = call "Read Instrument.lvclass.vi"("error in (no error)"=w7019, "S4ACS_GUI in"=w7020) -> ("error out"=w7039:errorcluster, "Instrument.lvclass"=w7041:refnum<class "Instrument.lvclass">, "S4ACS_GUI out"=w7040:refnum<class "S4GUI.lvclass">)  [unwired: 7 in]
            n2903 = call "Read WPROT.vi"("error in (no error)"=w7039, "Instrument in"=w7041) -> ("error out"=w7034:errorcluster, "Opt_Selector.lvclass"=w7037:refnum<class "Opt_Selector.lvclass">, "Instrument out"=w7042:refnum<class "Instrument.lvclass">)  [unwired: 7 in]
            n2904 = call-dynamic "Read sequencia_ant.vi"("error in (no error)"=w7034, "Opt_Selector in"=w7037) -> ("error out"=w7033:errorcluster, "sequencia_ant"=w7035:u16, "Opt_Selector out"=w7036:refnum<class "Opt_Selector.lvclass">)  [unwired: 7 in]
            n2905 = call-dynamic "Write sequencia.vi"("error in (no error)"=w7033, "sequencia"=w7035, "Opt_Selector in"=w7036) -> ("error out"=w7028:errorcluster, "Opt_Selector out"=w7029:refnum<class "Opt_Selector.lvclass">)  [unwired: 7 in]
            n2906 = call-dynamic "Read State Machine.vi"("error in (no error)"=w7028, "Device in"=w7029) -> ("error out"=w7031:errorcluster, "State Machine.lvclass"=w7026:refnum<class "State Machine.lvclass">, "Device out"=w7027:refnum<class "Opt_Selector.lvclass">)  [unwired: 7 in]
            n2907 = call "Next State.vi"("error in (no error)"=w7031, "New_State"=10, "State Machine in"=w7026) -> ("error out"=w7030:errorcluster, "State Machine out"=w7025:refnum<class "State Machine.lvclass">)  [unwired: 7 in]
            n2908 = call-dynamic "Write State Machine.vi"("error in (no error)"=w7030, "State Machine.lvclass"=w7025, "Device in"=w7027) -> ("error out"=w7024:errorcluster, "Device out"=w7023:refnum<class "Opt_Selector.lvclass">)  [unwired: 7 in]
